vi "SGUI Set Single Real By Label.vi"(6 "error in":errorcluster, 8 "label (empty)":string, 9 "format (empty)":string, 10 "value (none)":dbl=nan) -> (7 "error out":errorcluster, 11 "control reference out":refnum<vi>)   [LabVIEW 2020, in "varilib.lvlib"]
doc: "This VI sets value and format of numeric control designated by label name string. If empty format string is entered, format stays unchanged. If NaN value is entered, the value is not modified. \n\nThi VI ignores input errors (will execute anyway) however will generate error if any of the named controls is not found or writting to it fails (invalid type of control)."
uses:
  varilib.lvlib
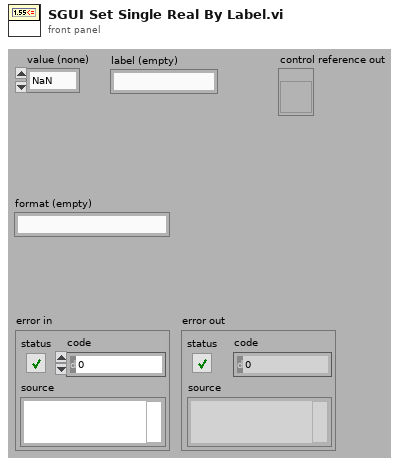
[diagram p1: front panel]
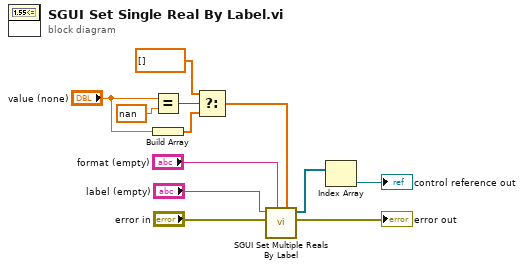
[diagram p0: block diagram]
diagram:
  n1 = Equal?(x="value (none)", y=nan) -> (x = y?=w6:bool)
  n2 = Build Array("value (none)") -> (w4:dbl[])
  n3 = Select(t=dbl[] [], s=w6, f=w4) -> (s? t:f=w2:dbl[])
  n4 = call "SGUI Set Multiple Reals By Label.vi"("error in"="error in", "labels (empty)"="label (empty)", "format (empty)"="format (empty)", "numbers (empty)"=w2) -> ("error out"=→"error out":errorcluster, "control references out"=w9:refnum<vi>[])  [unwired: 6 in]
  n5 = Index Array(array=w9) -> (element=→"control reference out":refnum<vi>)  [unwired: 1 in]
